vi "Handle Variable Header.vi"(8 "error in (no error)":errorcluster, 10 "Incoming Packets":u8[](array[numeric]) format="%08b", 11 "CONNACK in":refnum<class "CONNACK.lvclass">) -> (0 "error out":errorcluster, 1 "Variable Header Complete?":bool=TRUE, 2 "Remaining Packets":u8[](array[numeric]) format="%08b", 3 "CONNACK out":refnum<class "CONNACK.lvclass">)   [LabVIEW 2013, in "CONNACK.lvclass"]
uses:
  CONNACK.lvclass
  ControlPacket/ControlPacket.lvclass/ControlPacket.ctl
  ControlPacket/ControlPacket.lvclass
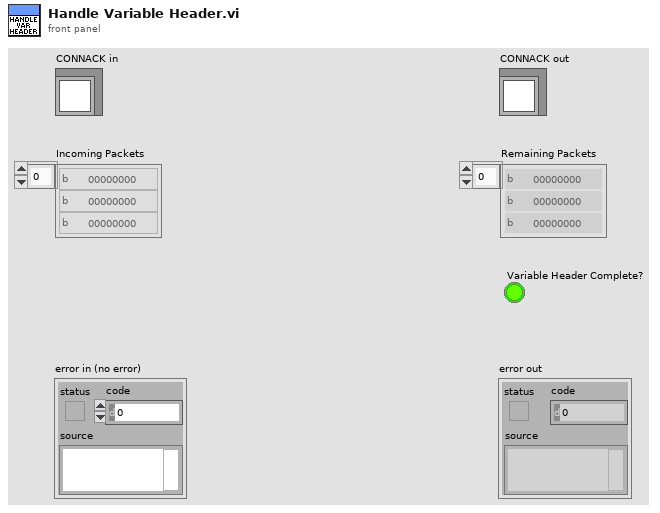
[diagram p1: front panel]
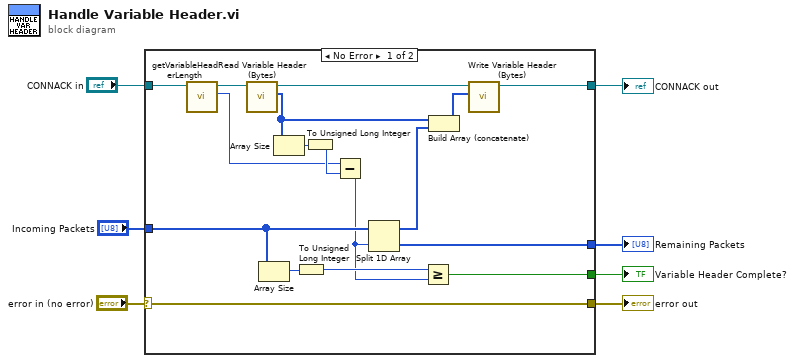
[diagram p0: block diagram]
diagram:
  n1 = case shown="No Error" "error in (no error)" {
    selector: "error in (no error)" -> [w9 w25]
    tunnel: "CONNACK in" -> [w22 w27]
    tunnel: "Incoming Packets" -> [w16 w26]
    tunnel: [w12 _] -> w2
    tunnel: [w11 w26] -> w3
    tunnel: [w10 w27] -> w4
    tunnel: [w9 w25] -> w1
    frame No Error {
      n2 = call-dynamic "getVariableHeaderLength.vi"("CONNACK in"=w22) -> ("VariableHeader size"=w8:u32, "CONNACK out"=w24:refnum<class "CONNACK.lvclass">)  [unwired: 8 in, 1 out]
      n3 = call "Read Variable Header (Bytes).vi"("ControlPacket in"=w24) -> ("Variable Header (Bytes)"=w20:u8[], "ControlPacket out"=w23:refnum<class "CONNACK.lvclass">)  [unwired: 9 in]
      n4 = Array Size(array=w16) -> (size(s)=w15:i32)
      n5 = Array Size(array=w20) -> (size(s)=w21:i32)
      n6 = To Unsigned Long Integer(number=w15) -> (unsigned 32bit integer=w14:u32)
      n7 = To Unsigned Long Integer(number=w21) -> (unsigned 32bit integer=w17:u32)
      n8 = Subtract(x=w8, y=w17) -> (x-y=w13:u32)
      n9 = Split 1D Array(array=w16, index=w13) -> (first subarray=w19:u8[], second subarray=w11:u8[])
      n10 = Greater Or Equal?(x=w14, y=w13) -> (x >= y?=w12:bool)
      n11 = Build Array (concatenate)(w20, w19) -> (w18:u8[])
      n12 = call "Write Variable Header (Bytes).vi"("Variable Header (Bytes)"=w18, "ControlPacket in"=w23) -> ("ControlPacket out"=w10:refnum<class "CONNACK.lvclass">)  [unwired: 9 in]
    }
    frame Error {
    }
  }
  "error out" <- w1
  "CONNACK out" <- w4
  "Remaining Packets" <- w3
  "Variable Header Complete?" <- w2
